vi "homework2.2.vi"() -> ()   [LabVIEW 2017]
panel:
  out "注册":bool
  in  "簇":cluster{"姓名":string, "学号":dbl, "注册":bool}
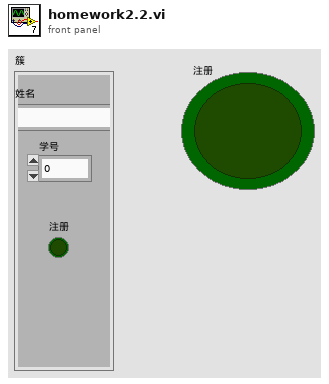
[diagram p1: front panel]
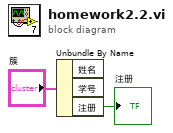
[diagram p0: block diagram]
diagram:
  n1 = Unbundle By Name("簇") -> ("注册"=→"注册":bool)  [unwired: 2 out]
